vi "Adjust FIFO Size.vi"(8 "error in (no error)":errorcluster, 10 "New FIFO Instance Config":T1 {"Custom Data" format="%.0x"}, 11 "CIF_CIPC_Chn in":refnum<class "CIF_CIPC_Chn.lvclass">) -> (0 "error out":errorcluster, 3 "CIF_CIPC_Chn out":refnum<class "CIF_CIPC_Chn.lvclass">)   [LabVIEW 2021, in "CIF_CIPC_Chn.lvclass"]
uses:
  CIF_CIPC_Chn.lvclass
  D:/dev/Packages/CIF_Channels_Core/src/CIFChannels/CIFChannels.lvclass
  ChannelCommon/typedef/New FIFO Instance Configuration.ctl
  CIF_CIPC_Chn.lvclass/CIF_CIPC_Chn.ctl
  CIFChannels/CIFChannels.lvclass/CIFChannels.ctl
  ChannelCommon/typedef/Errors.ctl
  CIFChannels/Typedef/Direction.ctl
  CIFChannels/Accessors/Read Channel State.vi
  CIFChannels/Accessors/Read Name.vi
  CIFChannels/Accessors/Read Custom Config Data.vi
  <vilib>/CIF Foundation/CIF CIPC/SubVIs/Check Error.vi
  <vilib>/CIF Foundation/CIF CIPC/SubVIs/Get dll Path.vi
  <vilib>/CIF Foundation/CIF Utilities/Errors/Append Error Location.vi
  <vilib>/CIF Foundation/CIF Utilities/DataTypes/Flatten Unflatten/Unflatten U64.vi
  <vilib>/CIF Foundation/CIF Utilities/DataTypes/Flatten Unflatten/Flatten U64.vi
  <vilib>/Utility/error.llb/Trim Whitespace.vi
  <vilib>/Utility/error.llb/Error Cluster From Error Code.vi
  <vilib>/CIF Foundation/CIF CIPC/CIF_NI_CIPC.lvlib
  CIFChannels/CIFChannels.lvclass
  ChannelCommon/ChannelCommon.lvlib
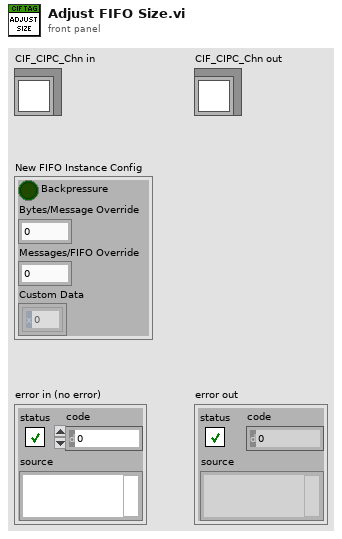
[diagram p1: front panel]
types:
  T1 = typedef "ChannelCommon.lvlib/New FIFO Instance Configuration.ctl" = cluster{"Backpressure":bool, "Bytes/Message Override":u32, "Messages/FIFO Override":u32, "Custom Data":u8[]}
  T2 = typedef "ChannelCommon.lvlib/Errors.ctl" = enum16{"gRPC Server Not Found", "Duplicate Channel", "Missing Channel", "Incorrect Type", "Flatten Error", "Unflatten Data", "Channel Length", "Plugin Connection", "gRPC Server Connection", "FIFO Unflatten", "Required Override", "Remove Not Found", "Multi Sub Not Supported", "Primary Already Connected", "Backpressure Not Supported", "Unable to Increase Buffer"}
  T3 = typedef "CIFChannels.lvclass/Direction.ctl" = enum16{"Publisher", "Subscriber"}
  T4 = typedef "CIFChannels.lvclass/Channel State.ctl" = enum16{"Creating", "Disconnected", "Connecting", "Connected", "Destroyed"}
  T5 = typedef "CIF_NI_CIPC.lvlib/Info Size.ctl" = cluster{"Max Element Size":u32, "Number of Elements":u32, "Elements in Memory":u32, "Frame Size":u32, "Order of Frame Size":u32, "Buffer Size":u32, "Order of Buffer Size":u32}
  T6 = typedef "ChannelCommon.lvlib/FIFO Config.ctl" = cluster{"Max Bytes/Msg":u64, "Max Msg/FIFO":u64, "Flags":u64, "Custom Data":u8[]}
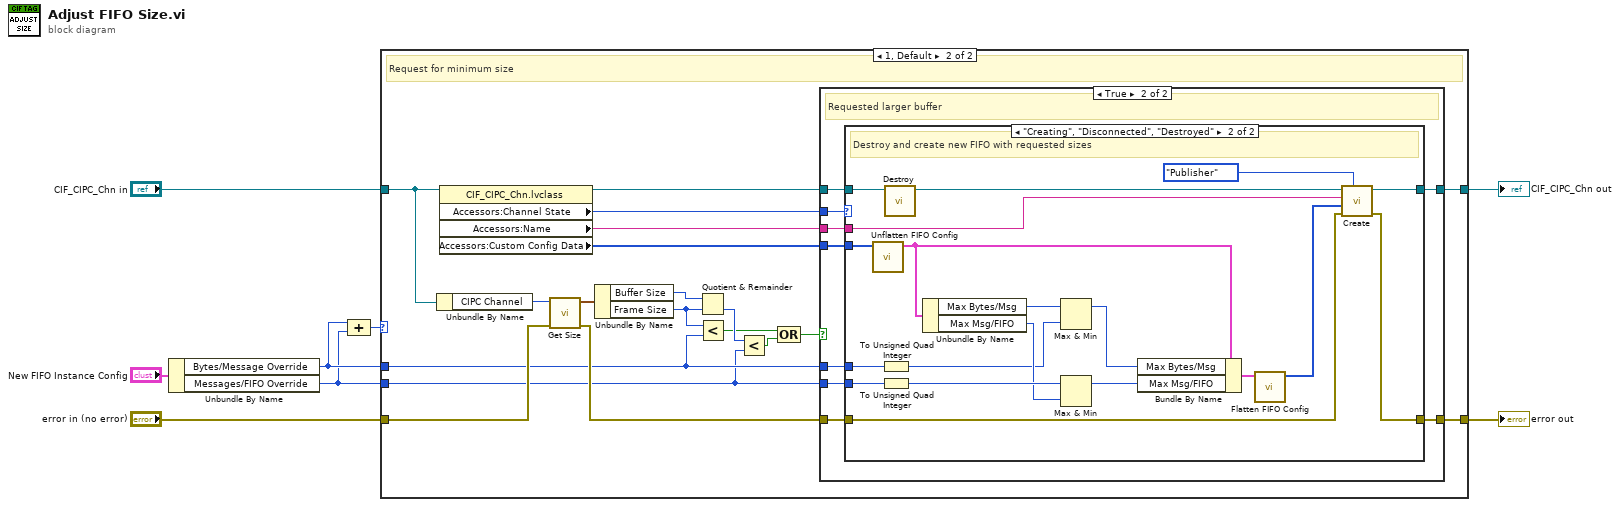
[diagram p0: block diagram]
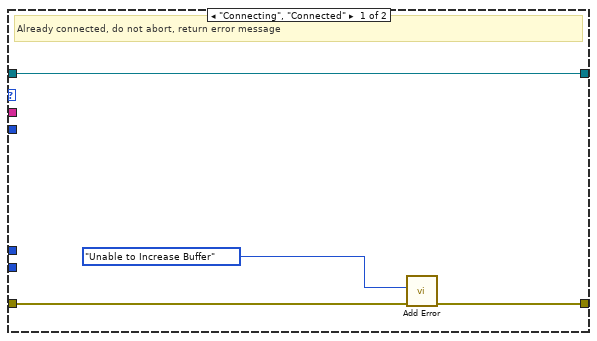
[diagram p4: hidden frame]
diagram:
  n1 = Unbundle By Name("New FIFO Instance Config") -> ("Bytes/Message Override"=w4:u32, "Messages/FIFO Override"=w3:u32)
  n2 = Compound Arithmetic op=ADD(w4, w3) -> (w5:u32)
  n3 = case shown="1, Default" w5 {
    tunnel: [w10 w22] -> w7
    tunnel: "CIF_CIPC_Chn in" -> [w10 w18]
    tunnel: w4 -> [_ w12]
    tunnel: w3 -> [_ w11]
    tunnel: "error in (no error)" -> [w9 w21]
    tunnel: [w9 w19] -> w1
    frame 0 {
      # "No request for custom FIFO size"
    }
    frame 1, Default {
      # "Request for minimum size"
      n4 = Unbundle By Name(w18) -> ("CIPC Channel"=w29:u64)
      n5 = property class="CIF_CIPC_Chn.lvclass"(reference=w18) -> (reference out=w17:refnum<class "CIF_CIPC_Chn.lvclass">, "Accessors:Channel State"=w16:T4, "Accessors:Name"=w15:string, "Accessors:Custom Config Data"=w14:u8[])  [unwired: 1 in, 1 out]
      n6 = call <vilib>:"Get Size.vi"("error in (no error)"=w21, "CIPC Reference"=w29) -> ("error out"=w20:errorcluster, "Size Info"=w28:T5)  [unwired: 8 in]
      n7 = Unbundle By Name(w28) -> ("Buffer Size"=w13:u32, "Frame Size"=w27:u32)
      n8 = Quotient & Remainder(x=w13, y=w27) -> (floor(x/y)=w26:u32)  [unwired: 1 out]
      n9 = Less?(x=w27, y=w12) -> (x < y?=w25:bool)
      n10 = Less?(x=w26, y=w11) -> (x < y?=w24:bool)
      n11 = Compound Arithmetic op=OR(w25, w24) -> (w23:bool)
      n12 = case shown="True" w23 {
        tunnel: w17 -> [w31 w39]
        tunnel: [w31 w37] -> w22
        tunnel: w20 -> [w30 w38]
        tunnel: [w30 w32] -> w19
        tunnel: w16 -> [_ w40]
        tunnel: w15 -> [_ w36]
        tunnel: w14 -> [_ w35]
        tunnel: w12 -> [_ w34]
        tunnel: w11 -> [_ w33]
        frame False {
          # "Existing buffer is large enough, no action."
        }
        frame True {
          # "Requested larger buffer"
          n13 = case shown="\"Creating\", \"Disconnected\", \"Destroyed\"" w40 {
            tunnel: w39 -> [w44 w63]
            tunnel: w38 -> [w42 w54]
            tunnel: [w44 w52] -> w37
            tunnel: w36 -> [_ w60]
            tunnel: w35 -> [_ w59]
            tunnel: w34 -> [_ w57]
            tunnel: w33 -> [_ w58]
            tunnel: [w41 w53] -> w32
            frame "Connecting", "Connected" {
              # "Already connected, do not abort, return error message"
              n14 = call "Add Error.vi"("error in (no error)"=w42, "Error"=Errors."Unable to Increase Buffer") -> ("error out"=w41:errorcluster)  [unwired: 9 in]
            }
            frame "Creating", "Disconnected", "Destroyed" {
              # "Destroy and create new FIFO with requested sizes"
              n15 = call "Unflatten FIFO Config.vi"("Flattened Data in"=w59) -> ("FIFO Config out"=w51:T6)  [unwired: 9 in, 1 out]
              n16 = To Unsigned Quad Integer(1:w57) -> (0:w46:u64)
              n17 = To Unsigned Quad Integer(1:w58) -> (0:w49:u64)
              n18 = call-dynamic "Destroy.vi"("CIFTag in"=w63) -> ("CIFTag out"=w62:refnum<class "CIF_CIPC_Chn.lvclass">)  [unwired: 9 in, 1 out]
              n19 = Unbundle By Name(w51) -> ("Max Bytes/Msg"=w47:u64, "Max Msg/FIFO"=w48:u64)
              n20 = Max & Min(x=w47, y=w46) -> (max(x,y)=w45:u64)  [unwired: 1 out]
              n21 = Max & Min(x=w49, y=w48) -> (max(x,y)=w50:u64)  [unwired: 1 out]
              n22 = Bundle By Name(cluster=w51, "Max Bytes/Msg"=w45, "Max Msg/FIFO"=w50) -> (w56:T6)
              n23 = call "Flatten FIFO Config.vi"("FIFO Config in"=w56) -> ("Flattened FIFO Config"=w55:u8[])  [unwired: 10 in]
              n24 = call-dynamic "Create.vi"("Direction"=Direction."Publisher", "error in (no error)"=w54, "Custom Config Data"=w55, "Name"=w60, "CIFChannels in"=w62) -> ("error out"=w53:errorcluster, "CIFChannels out"=w52:refnum<class "CIF_CIPC_Chn.lvclass">)  [unwired: 5 in]
            }
          }
        }
      }
    }
  }
  "error out" <- w1
  "CIF_CIPC_Chn out" <- w7
